vi "DigitalOutputToDevice.vi"(8 "error in (no error)":errorcluster, 11 "TesteractHAL_DigitalIO In":refnum<class "TesteractHAL_DigitalOutput.lvclass">) -> (0 "error out":errorcluster, 3 "TesteractHAL_Device Out":refnum<class "TesteractHAL_Device.lvclass">)   [LabVIEW 2017, in "TesteractHAL_DigitalOutput.lvlib" / "TesteractHAL_DigitalOutput.lvclass"]
doc: "Converts a DigitalIO object into a Device object.\n\nIgnores errors and just passes them through."
uses:
  TesteractHAL_DigitalOutput.lvclass
  Program Files (x86)/Testeract/HWLib/HAL/Device/TesteractHAL_Device.lvlibp/TesteractHAL_Device.lvclass
  C:/Program Files (x86)/Testeract/HWLib/HAL/Device/TesteractHAL_Device.lvlibp/TesteractHAL_Device.lvclass
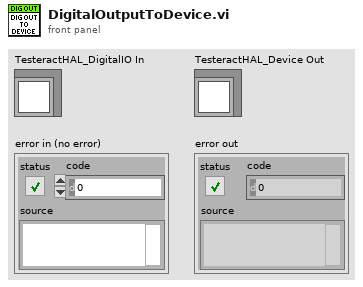
[diagram p1: front panel]
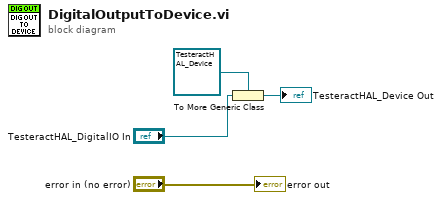
[diagram p0: block diagram]
diagram:
  n1 = To More Generic Class(target class=refnum<class "TesteractHAL_Device.lvclass"> refnum ("TesteractHAL_Device.lvlibp:TesteractHAL_Device.lvclass"), reference="TesteractHAL_DigitalIO In") -> (generic class reference=→"TesteractHAL_Device Out":refnum<class "TesteractHAL_Device.lvclass">)
  "error out" <- "error in (no error)"
